vi "Scale and Checksum.vi"(0 "Raw Data":bool[](array[boolean])=[FALSE, FALSE, FALSE, FALSE, FALSE, FALSE, FALSE, FALSE, FALSE, FALSE, FALSE, FALSE, FALSE, FALSE, FALSE, FALSE, FALSE, FALSE, FALSE, FALSE, FALSE, FALSE, FALSE, FALSE, FALSE, FALSE, FALSE, FALSE, FALSE, FALSE, FALSE, FALSE, FALSE, FALSE, FALSE, FALSE, FALSE, FALSE, FALSE, FALSE]) -> (4 "Temperature (°C)":u8, 8 "Humidity (%)":u8, 15 "Valid?":bool)   [LabVIEW 2014, in "DHT11 (FPGA).lvlib"]
uses:
  DHT11 (FPGA).lvlib
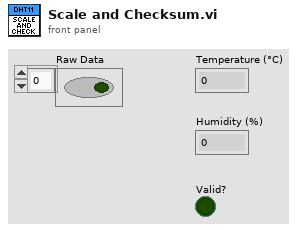
[diagram p1: front panel]
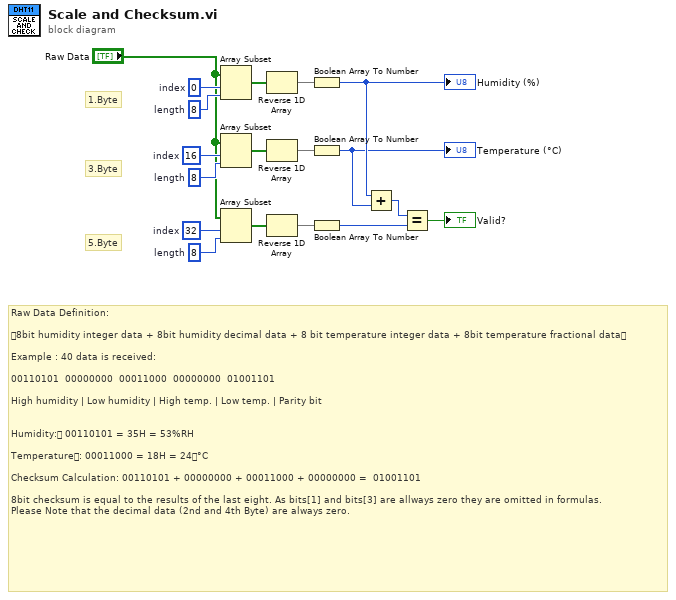
[diagram p0: block diagram]
diagram:
  w13 = 8  # length
  w14 = 32  # index
  w16 = 8  # length
  w15 = 16  # index
  w17 = 8  # length
  w18 = 0  # index
  # "5.Byte"
  # "3.Byte"
  # "1.Byte"
  # "Raw Data Definition:\n\n8bit humidity integer data + 8bit humidity decimal data + 8 bit temperature integer data + 8bit temperature fractional data\n\nExample : 40 data is received:\n\n00110101  00000000  00011000  00000000  01001101\n\nHigh humidity | Low humidity | High temp. | Low temp. | Parity bit\n\n\nHumidity: 00110101 = 35H = 53%RH\n\nTemperature: 00011000 = 18H = 24°C\n\nChecksum Calculation: 00110101 + 00000000 + 00011000 + 00000000 =  01001101\n\n8bit checksum is equal to the results of the last eight. As bits[1] and bits[3] are allways zero they are omitted in formulas. \nPlease Note that the decimal data (2nd and 4th Byte) are always zero."
  n1 = Array Subset(array="Raw Data", index=w18, length=w17) -> (w12:bool[])
  n2 = Array Subset(array="Raw Data", index=w15, length=w16) -> (w10:bool[])
  n3 = Array Subset(array="Raw Data", index=w14, length=w13) -> (w8:bool[])
  n4 = Reverse 1D Array(array=w12) -> (reversed array=w11:bool[])
  n5 = Reverse 1D Array(array=w10) -> (reversed array=w9:bool[])
  n6 = Reverse 1D Array(array=w8) -> (reversed array=w7:bool[])
  n7 = Boolean Array To Number(Boolean array=w11) -> (number=w6:u8)
  "Humidity (%)" <- w6
  n8 = Boolean Array To Number(Boolean array=w9) -> (number=w5:u8)
  "Temperature (°C)" <- w5
  n9 = Boolean Array To Number(Boolean array=w7) -> (number=w3:u8)
  n10 = Add(x=w6, y=w5) -> (x+y=w4:u8)
  n11 = Equal?(x=w4, y=w3) -> (x = y?=→"Valid?":bool)
